vi "Configure Output Power.vi"(8 "error in (no error)":errorcluster, 10 "Output Power [dBm]":dbl, 11 "PSG-MXG in":refnum<class "PSG-MXG.lvclass">) -> (0 "error out":errorcluster, 3 "PSG-MXG out":refnum<class "PSG-MXG.lvclass">)   [LabVIEW 2020, in "PSG-MXG.lvclass"]
uses:
  PSG-MXG.lvclass
  C:/Sandbox/Git_Sandbox/WiSpry Test Framework source code (LV20)/WiSpry Test Framework/Instruments/Instrument.lvclass
  C:/Sandbox/Git_Sandbox/WiSpry Test Framework source code (LV20)/WiSpry Test Framework/Instruments/Signal Generator/Signal Generator.lvclass
  Instrument.lvclass/Instrument.ctl
  Signal Generator.lvclass/Signal Generator.ctl
  Instrument.lvclass
  Signal Generator.lvclass
  <instrlib>/Agilent PSG MXG Series/Agilent PSG MXG Series.lvlib
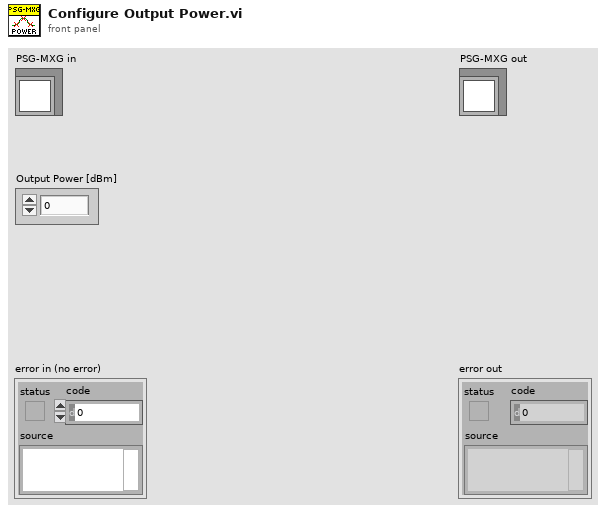
[diagram p1: front panel]
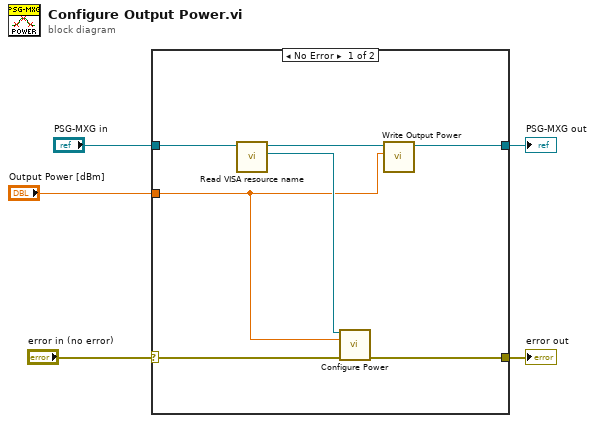
[diagram p0: block diagram]
diagram:
  n1 = case shown="No Error" "error in (no error)" {
    selector: "error in (no error)" -> [w9 w14]
    tunnel: "PSG-MXG in" -> [w12 w13]
    tunnel: [w8 w14] -> w3
    tunnel: [w10 w13] -> w2
    tunnel: "Output Power [dBm]" -> [w6 _]
    frame No Error {
      n2 = call "Read VISA resource name.vi"("Instrument in"=w12) -> ("VISA resource name"=w7:refnum<visa-resource-name>, "Instrument out"=w11:refnum<class "PSG-MXG.lvclass">)  [unwired: 9 in]
      n3 = call <instrlib>:"Configure Power.vi"("VISA resource name"=w7, "Power (-130 dBm)"=w6, "error in (no error)"=w9) -> ("error out"=w8:errorcluster)  [unwired: 11 in, 1 out]
      n4 = call "Write Output Power.vi"("Output Power"=w6, "Signal Generator in"=w11) -> ("Signal Generator out"=w10:refnum<class "PSG-MXG.lvclass">)  [unwired: 9 in]
    }
    frame Error {
    }
  }
  "error out" <- w3
  "PSG-MXG out" <- w2
